vi "emi_About window.vi"(2 "Fade/Rise time s(0)":dbl, 9 "error in (no error)":errorcluster) -> (10 "error out":errorcluster)   [LabVIEW 2011]
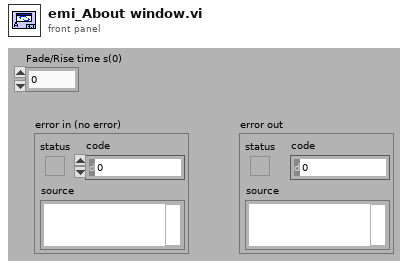
[diagram p1: front panel]
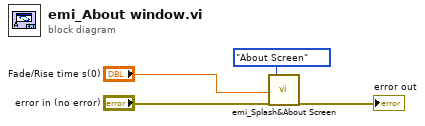
[diagram p0: block diagram]
diagram:
  n1 = call "emi_Splash&About Screen.vi"("Fade/Rise time s(0)"="Fade/Rise time s(0)", "error in (no error)"="error in (no error)", "Action"=enum16{"Start", "Update", "End", "About Screen"}."About Screen") -> ("error out"=→"error out":errorcluster)  [unwired: 16 in]
